vi "CamAcqu_WaitForTrigger.vi"(10 "Session in":T2, 11 "Image in":T1) -> (1 "Acquisition OK?":bool, 2 "Session Out":T2, 3 "Image  Out":T1)   [LabVIEW 2013]
uses:
  <vilib>/userdefined/High Color/IMAQdx.ctl
  <vilib>/vision/Image Controls.llb/IMAQ Image.ctl
  <vilib>/vision/NI_Vision_Development_Module.lvlib
  <vilib>/vision/driver/NI_Vision_Acquisition_Software.lvlib
panel:
  in  "error in":errorcluster
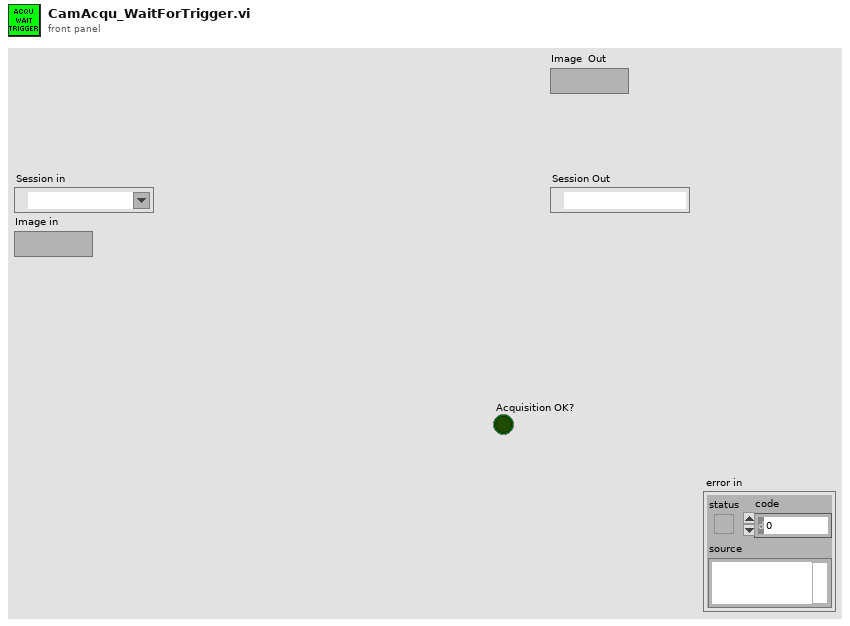
[diagram p1: front panel]
types:
  T1 = typedef "IMAQ Image.ctl" = refnum<image>
  T2 = typedef "IMAQdx.ctl" = refnum<k21>
  T3 = typedef "Image Type" = u32
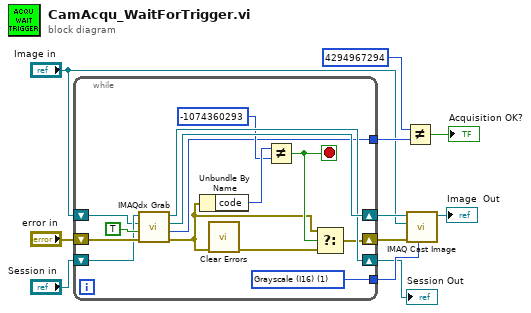
[diagram p0: block diagram]
diagram:
  n1 = while {
    tunnel: [w24] -> w11
    tunnel: [w12] -> w7
    shift-right: [w15] -> w6
    shift-left: "error in" -> [w22]
    shift-right: [w23] -> w10
    shift-left: "Image in" -> [w13]
    shift-right: [w21] -> w2
    shift-left: "Session in" -> [w14]
    stop <- w18 stop-if-true
    w24 = T3 1 items=["Grayscale (U8)", "Grayscale (I16)", "Grayscale (SGL)", "Complex (CSG)", "RGB (U32)", "HSL (U32)", "RGB (U64)", "Grayscale (U16)"] ("Image Type")
    n2 = call <vilib>:"IMAQdx Grab.vi"("error in"=w22, "Wait for Next Buffer? (Yes)"=TRUE, "Image In"=w13, "Session In"=w14) -> ("error out"=w17:errorcluster, "Buffer Number Out"=w12:u32, "Image Out"=w23:T1, "Session Out"=w21:T2)  [unwired: 4 out]
    n3 = Unbundle By Name(w17) -> ("code"=w20:i32)
    n4 = call <vilib>:"Clear Errors.vi"("error in (no error)"=w17) -> ("error out"=w16:errorcluster)  [unwired: 6 in]
    n5 = Not Equal?(x=w20, y=-1074360293 ("code 2")) -> (x != y?=w18:bool)
    n6 = Select(t=w17, s=w18, f=w16) -> (s? t:f=w15:errorcluster)
  }
  "Session Out" <- w2
  n7 = Not Equal?(x=u32 4294967294 ("Buffer Number Out"), y=w7) -> (x != y?=→"Acquisition OK?":bool)
  n8 = call "IMAQ Cast Image"("Image Type"=w11, "error in (no error)"=w6, "Image Dst"="Image in", "Image Src"=w10) -> ("Image Dst Out"=→"Image  Out":T1)  [unwired: 6 in, 1 out]
